vi "Unregister All.vi"(8 "error in (no error)":errorcluster) -> (0 "error out":errorcluster, 3 "loggers":refnum<class "Logger.lvclass">[](array[class]))   [LabVIEW 2018, in "GLog.lvlib" / "Registry.lvlib"]
uses:
  Registry.lvlib
  api/logger_class/Logger.lvclass
  Registry Actions.ctl
  reuse_library/Utilities/Utilities.lvlib
panel:
  # "Connector Pane"
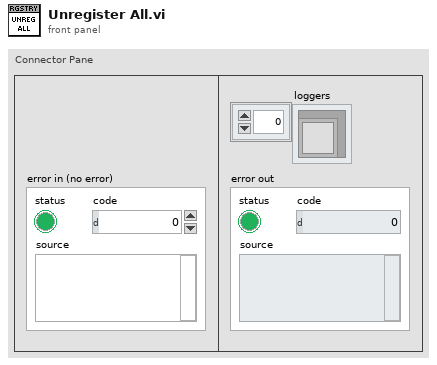
[diagram p1: front panel]
types:
  T1 = typedef "GLog.lvlib/Registry.lvlib/Registry Actions.ctl" = enum16{"Register", "Log", "Enable", "Enable All", "Disable", "Disable All", "List", "Unregister", "Unregister All", "Shutdown"}
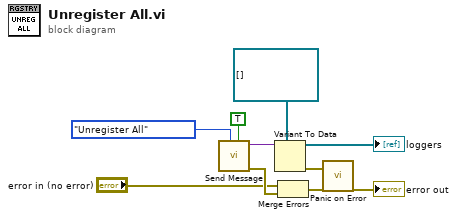
[diagram p0: block diagram]
diagram:
  n1 = call "Send Message.vi"("return data? (F)"=TRUE, "action"=Registry_Actions."Unregister All") -> ("error out"=w6:errorcluster, "return data"=w8:variant)  [unwired: 8 in]
  n2 = Variant To Data(type=refnum<class "Logger.lvclass">[] [] ("Array"), Variant=w8) -> (data=→"loggers":refnum<class "Logger.lvclass">[], error out=w3:errorcluster)  [unwired: 1 in]
  n3 = Merge Errors("error in (no error)", w6) -> (→"error out":errorcluster)
  n4 = call "Panic on Error.vi"("error in (no error)"=w3) -> ()  [unwired: 3 in]
